vi "forward.vi"   [LabVIEW 2012, in "sumobot 18.lvrbt"]
uses:
  sumobot 18.lvrbt
  <vilib>/NXT/Block Support/NXT_OutputPort.ctl
  <vilib>/NXT/Dual Mode Library/Waits/Wait_Num.vi
  <vilib>/NXT/NXTIO Xnodes/NXTIONodeSubVIs/NXTMoveMotors.vi
  <vilib>/NXT/NXTIO Xnodes/NXTIONodeSubVIs/LEGOStopAllMotors.vi
  <vilib>/NXT/Subs/LVHSConnector.ctl
  <vilib>/NXT/NXTIO Xnodes/AddressXNode/NXTIOAddress.xnode
  <vilib>/NXT/NXTIO Xnodes/NXTIOXNode/NXTIO.xnode
  <vilib>/NXT/LegoClasses/BrickReference/BrickReference.lvclass
types:
  T1 = typedef "NXT_OutputPort.ctl" = u8
  T2 = typedef "LVHSConnector.ctl" = refnum<class "BrickReference.lvclass">
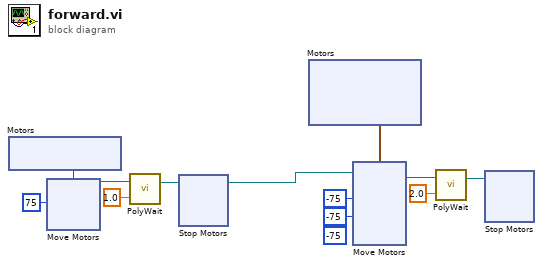
[diagram p0: block diagram]
diagram:
  (unwired) i8 -75 ("Power/Speed 2")
  n1 = xnode "Motors"() -> ("Motor"=w12:T1)
  n2 = xnode "Move Motors"("Power/Speed 1"=i8 75, "Motors"=w12) -> ("NXT/EV3"=w10:T2)  [unwired: 1 in]
  n3 = call-poly <vilib>:"PolyWait.vi"("Time (1 sec)"=sgl 1.0, "NXT/EV3"=w10) -> ("NXT/EV3"=w8:T2)  [unwired: 2 in]
  n4 = xnode "Stop Motors"("NXT/EV3"=w8) -> ("NXT/EV3"=w2:T2)  [unwired: 1 in]
  n5 = xnode "Motors"() -> ("Motor"=w7:cluster{"Port":T1, "Port":T1, "Port":T1})
  n6 = xnode "Move Motors"("Power/Speed 2"=i8 -75, "Power/Speed 1"=i8 -75, "Motors"=w7, "NXT/EV3"=w2) -> ("NXT/EV3"=w5:T2)  [unwired: 1 in]
  n7 = call-poly <vilib>:"PolyWait.vi"("Time (1 sec)"=sgl 2.0, "NXT/EV3"=w5) -> ("NXT/EV3"=w3:T2)  [unwired: 2 in]
  n8 = xnode "Stop Motors"("NXT/EV3"=w3) -> ()  [unwired: 1 in, 1 out]
